vi "Sensirion SHT25 - VISA open.vi"(8 "Error In":errorcluster, 11 "VISA in":refnum<visa-resource-name>) -> (0 "Error Out":errorcluster, 3 "VISA out":refnum<visa-resource-name>)   [LabVIEW 2012]
uses:
  <vilib>/Instr/_visa.llb/VISA Configure Serial Port (Instr).vi
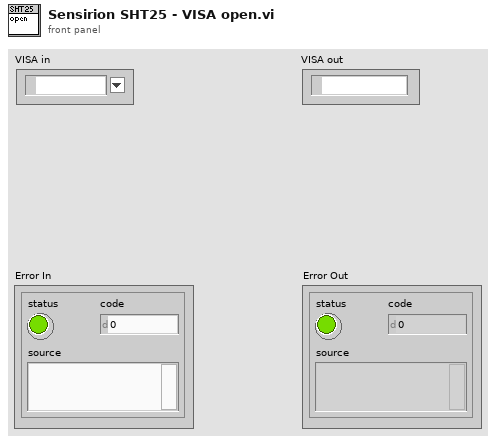
[diagram p1: front panel]
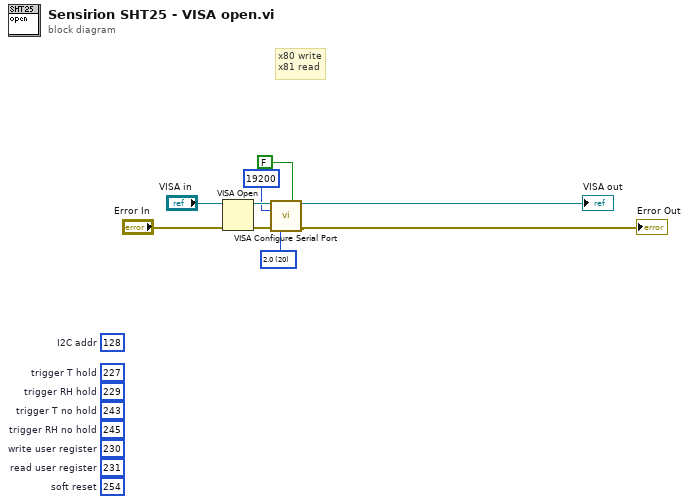
[diagram p0: block diagram]
diagram:
  (unwired) u8 254  # soft reset
  (unwired) u8 231  # read user register
  (unwired) u8 230  # write user register
  (unwired) u8 245  # trigger RH no hold
  (unwired) u8 243  # trigger T no hold
  (unwired) u8 229  # trigger RH hold
  w6 = u16 20 items=["1.0"=10, "1.5"=15, "2.0"=20] ("stop bits (10: 1 bit)")
  (unwired) u8 128  # I2C addr
  (unwired) u8 227  # trigger T hold
  # "x80 write\nx81 read"
  n1 = VISA Open(error in (no error)="Error In", VISA resource name="VISA in") -> (VISA resource name=w9:refnum<visa-resource-name>, error out=w8:errorcluster)  [unwired: 3 in]
  n2 = call-poly "VISA Configure Serial Port"("VISA resource name"=w9, "Enable Termination\nChar (T)"=FALSE ("Enable Termination\nChar (T)"), "baud rate (9600)"=u32 19200, "error in (no error)"=w8, "stop bits (10: 1 bit)"=w6) -> ("VISA resource name out"=→"VISA out":refnum<visa-resource-name>, "error out"=→"Error Out":errorcluster)  [unwired: 9 in]
